vi "Set WLAN LO Offset.vi"(0 "SG Reference":refnum<k15>, 5 "Carrier Frequency":dbl, 7 "LO Offset Settings":T1, 11 "error in (no error)":errorcluster) -> (4 "SG Reference out":refnum<k15>, 8 "LO Offset":dbl, 15 "error out":errorcluster)   [LabVIEW 2018, in "SG.lvlib"]
uses:
  SG.lvlib
  Typedefs/LO Offset Config.ctl
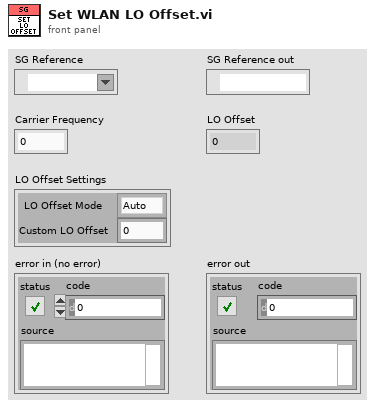
[diagram p1: front panel]
types:
  T1 = typedef "SG.lvlib/LO Offset Config.ctl" = cluster{"LO Offset Mode":enum16{"Auto", "Custom", "Disabled"}, "Custom LO Offset":dbl}
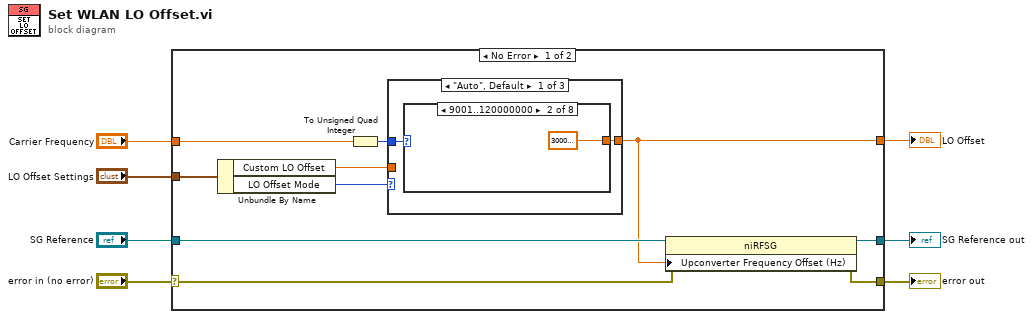
[diagram p0: block diagram]
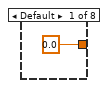
[diagram p2: hidden frame]
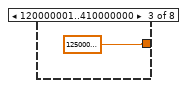
[diagram p3: hidden frame]
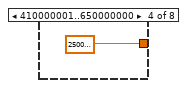
[diagram p4: hidden frame]
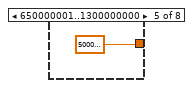
[diagram p5: hidden frame]
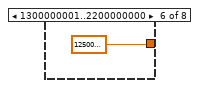
[diagram p6: hidden frame]
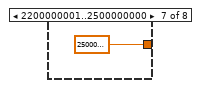
[diagram p7: hidden frame]
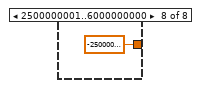
[diagram p8: hidden frame]
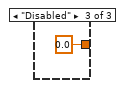
[diagram p10: hidden frame]
diagram:
  n1 = case shown="No Error" "error in (no error)" {
    selector: "error in (no error)" -> [w10 w31]
    tunnel: [w9 w31] -> w6
    tunnel: "SG Reference" -> [w17 w30]
    tunnel: [w16 w30] -> w4
    tunnel: [w14 _] -> w3
    tunnel: "LO Offset Settings" -> [w13 _]
    tunnel: "Carrier Frequency" -> [w8 _]
    frame No Error {
      n2 = Unbundle By Name(w13) -> ("Custom LO Offset"=w11:dbl, "LO Offset Mode"=w12:enum16{"Auto", "Custom", "Disabled"})
      n3 = To Unsigned Quad Integer(1:w8) -> (0:w15:u64)
      n4 = case shown="\"Auto\", Default" w12 {
        tunnel: w15 -> [w19 _ _]
        tunnel: [w18 w28 0.0 ("LO Offset")] -> w14
        tunnel: w11 -> [_ w28 _]
        frame "Auto", Default {
          n5 = case shown="9001..120000000" w19 {
            tunnel: [0.0 ("LO Offset") 30000000.0 ("LO Offset") 12500000.0 ("LO Offset") 25000000.0 ("LO Offset") 50000000.0 ("LO Offset") 125000000.0 ("LO Offset") 250000000.0 ("LO Offset") -250000000.0 ("LO Offset")] -> w18
            frame Default {
            }
            frame 9001..120000000 {
            }
            frame 120000001..410000000 {
            }
            frame 410000001..650000000 {
            }
            frame 650000001..1300000000 {
            }
            frame 1300000001..2200000000 {
            }
            frame 2200000001..2500000000 {
            }
            frame 2500000001..6000000000 {
            }
          }
        }
        frame "Custom" {
        }
        frame "Disabled" {
        }
      }
      n6 = property class="niRFSG"(reference=w17, error in=w10, "Upconverter Frequency Offset (Hz)"=w14) -> (reference out=w16:refnum<k15>, error out=w9:errorcluster)
    }
    frame Error {
    }
  }
  "error out" <- w6
  "SG Reference out" <- w4
  "LO Offset" <- w3
